vi "LC_BESS_Main.vi"() -> ()   [LabVIEW 2016]
uses:
  LabVIEW Data/MathScriptVIs/MCStatic_36913153632_b27534ebdc28079805a0f770a8a2da2a.vi
  <instcachedir>/0/MCStatic_36913153632_b27534ebdc28079805a0f770a8a2da2a_943E3674364E42B8AD23C55717B072BE.lvgen/MCStatic_36913153632_b27534ebdc28079805a0f770a8a2da2a_943E3674364E42B8AD23C55717B072BE_000.vi
  <vilib>/imath/engines/lvmath2/RunTimeEngine/BuiltInFunctions/abs/NIMS_abs(unsigned).vi
  <instcachedir>/0/NIMS_abs(unsigned)_CB0E2CC90712458C87FBF103B22FBEA1.lvgen/NIMS_abs(unsigned)_CB0E2CC90712458C87FBF103B22FBEA1_002.vi
  <vilib>/imath/engines/lvmath2/RunTimeEngine/NodeEndStatement/NIMS_NodeEndStatement_Output.vi
  <instcachedir>/0/NIMS_NodeEndStatement_Output_53EC0D466D134D7ABD903AC30B43404B.lvgen/NIMS_NodeEndStatement_Output_53EC0D466D134D7ABD903AC30B43404B_001.vi
  <vilib>/imath/engines/lvmath2/RunTimeEngine/ErrorHandling/NIMS_Finalize Error.vi
  <vilib>/ErrorRing/Error Ring.xnode
  BESS_LC/PIcontroller.m
panel:
  out "Waveform Chart":dbl[][](graph)=[[-0.0, 0.25, 0.0]]
  in  "BESS_Active_Power_Cmd 2":fxp<+/-,64,32>=0.25
  out "MGCC_to_BESS":dbl[](array[numeric])=[1.0, 0.0, 0.0, 0.0, 0.0, 0.0, 0.0] format="%#_6f"
  in  "p_mag":dbl=-1.0
  in  "i_mag":dbl=-1.0
  out "Waveform Chart 2":dbl(graph)
  out "BESS_Start_Stop_Cmd":bool
  out "error out 3":errorcluster
  out "error out 2":errorcluster
  out "BESS_Active_Power_Cmd":fxp<+/-,64,32>=0.25
  in  "Enable":bool=TRUE
  in  "p_in":dbl=0.5
  in  "i_in":dbl=0.2
  in  "p_an":dbl=0.2
  in  "i_an":dbl=0.05
  out "error out":errorcluster
  in  "BESS_Start_Stop":bool
  in  "BESS_Rective_Power_Cmd":fxp<+/-,64,32>=-1.0
  out "BESS_F":fxp<+/-,64,32>=59.92425537109375
  out "BESS_P":fxp<+/-,64,32>=0.000335693359375
  out "BESS_Q":fxp<+/-,64,32>=0.0039520263671875
  out "BESS_V":fxp<+/-,64,32>=0.0112762451171875
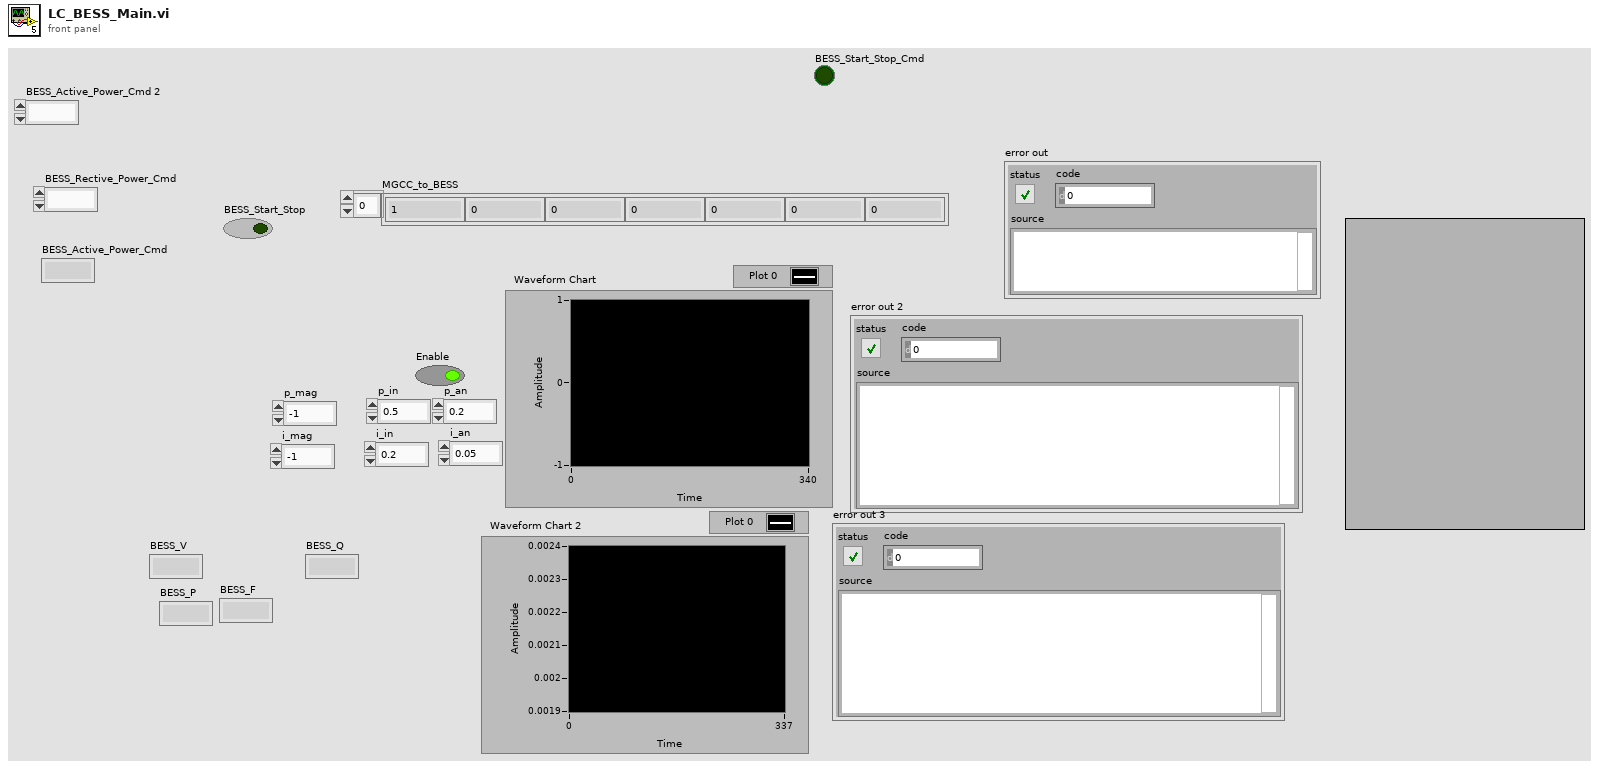
[diagram p1: front panel]
types:
  T1 = typedef "NI_Matrix.lvlib/RealMatrix.ctl" = dbl[][]
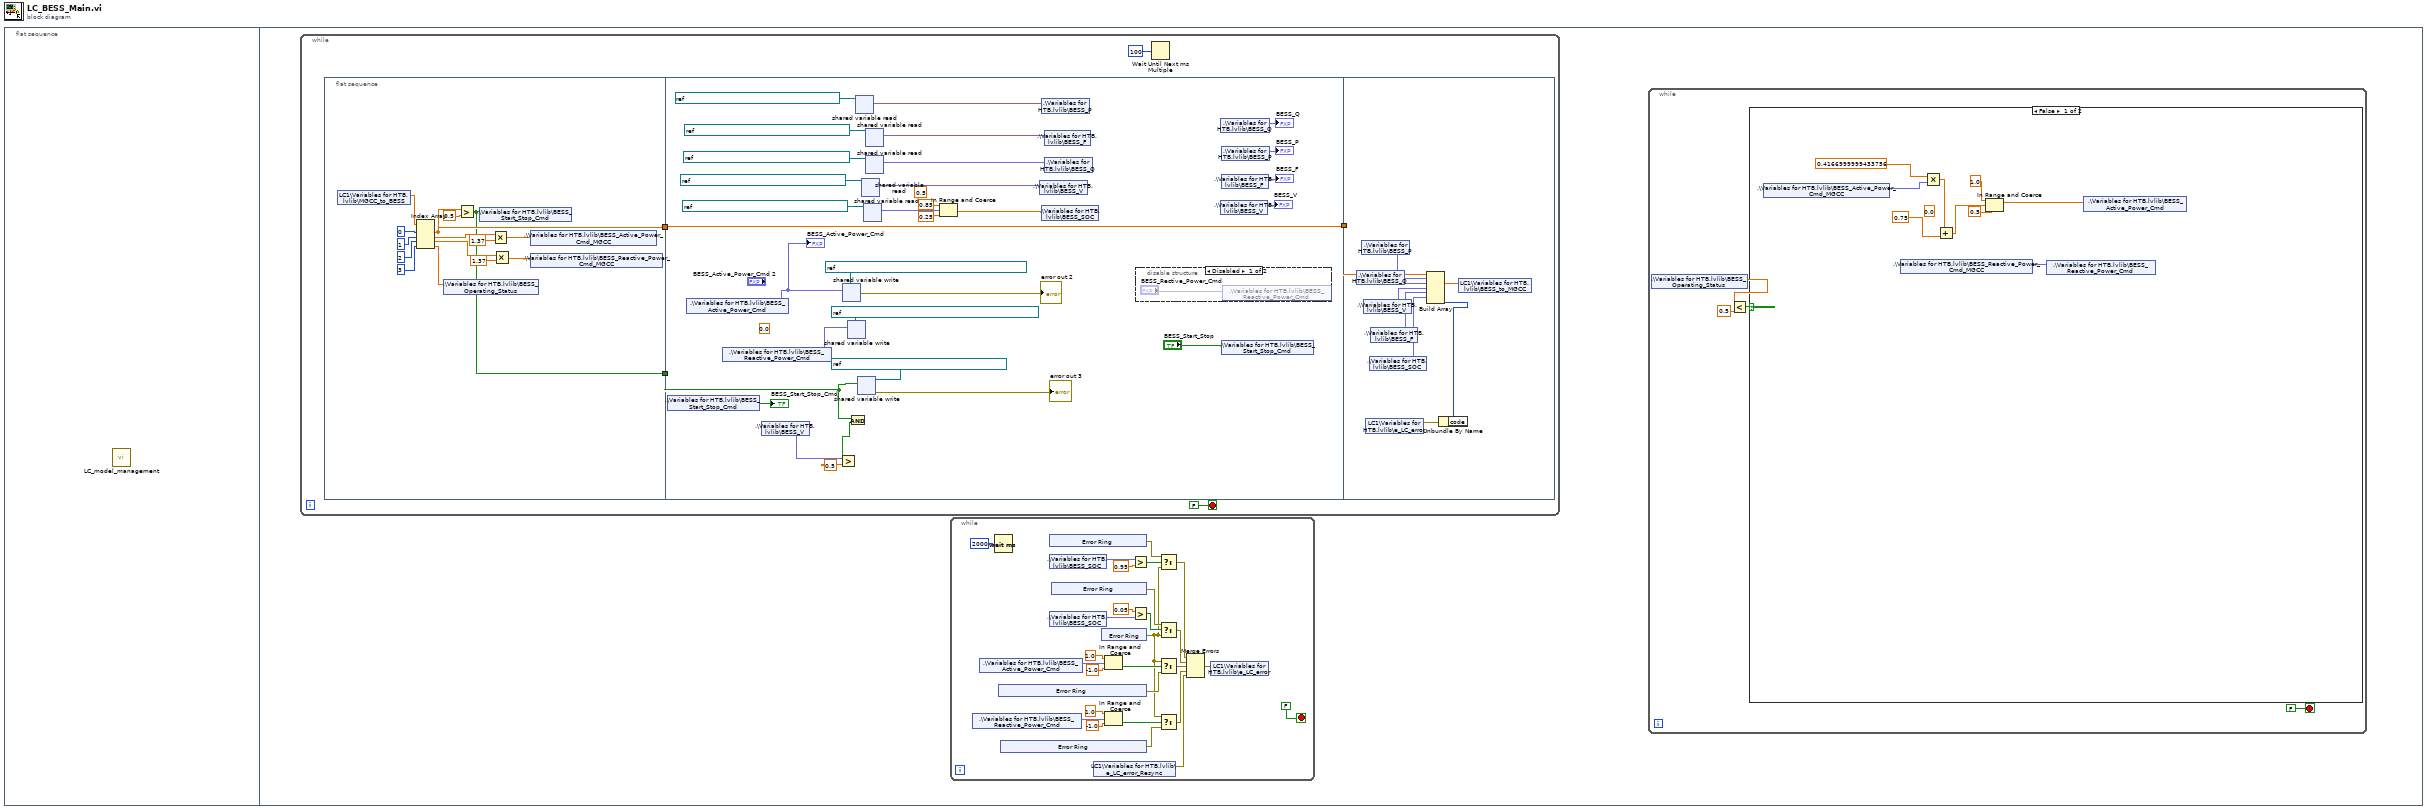
[diagram p0: block diagram]
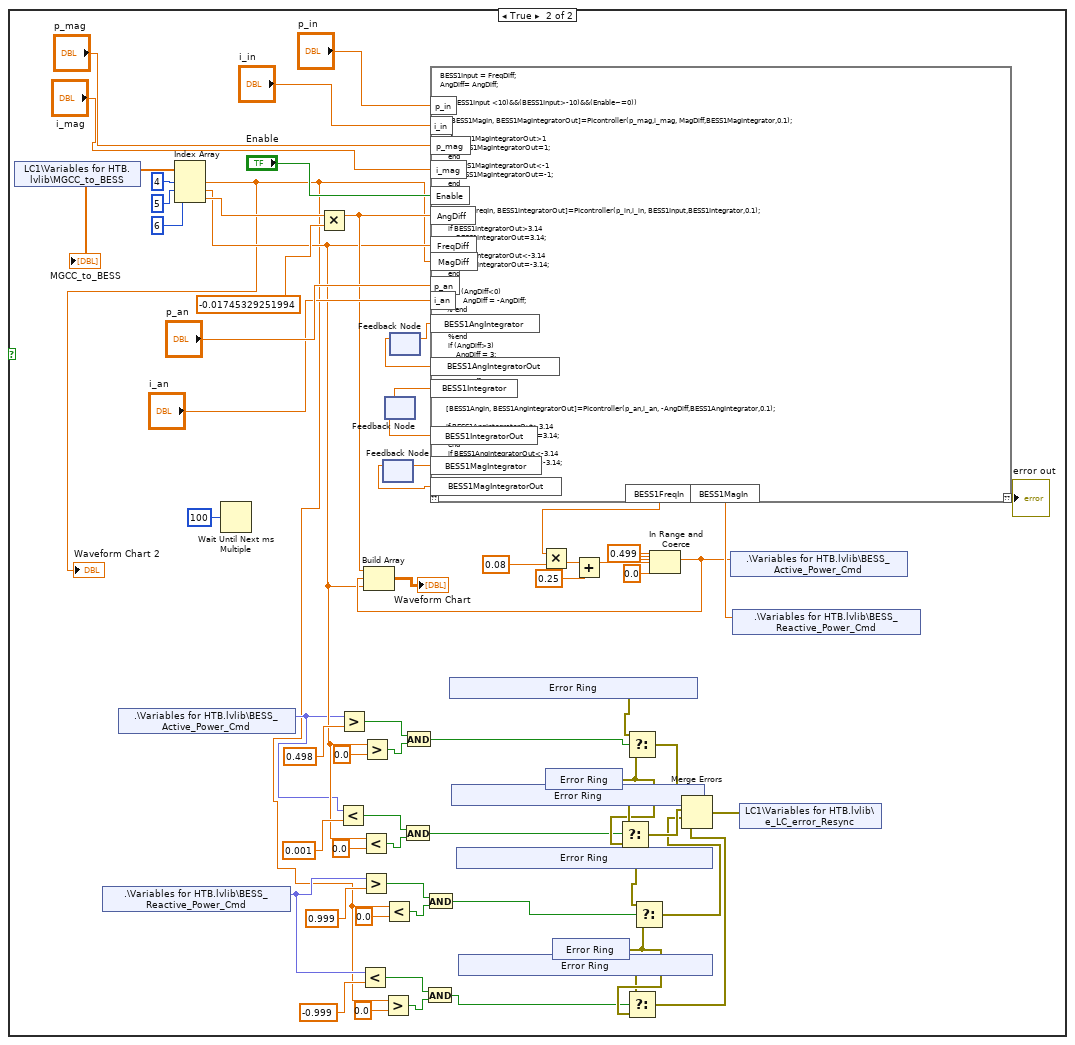
[diagram p2: hidden frame]
diagram:
  n1 = flat-sequence {
    frame #0 {
      n2 = call "LC_model_management.vi"() -> ()  [unwired: 12 in]
    }
    frame #1 {
      n3 = while {
        stop <- FALSE stop-if-true
        n4 = flat-sequence {
          tunnel: [w586] -> w573
          tunnel: [w583] -> w572
          tunnel: [w609] -> w574
          tunnel: w573 -> [w609]
          tunnel: w572 -> [w605]
          tunnel: w574 -> [w626]
          frame #0 {
            n5 = shared-variable "LC1\\Variables for HTB.lvlib\\MGCC_to_BESS"() -> (w591:dbl[])  [unwired: 1 in, 1 out]
            n6 = Index Array(array=w591, index #1=0 ("index"), index #2=1 ("index"), index #3=2 ("index"), index #4=3 ("index")) -> (element #1=w586:dbl, element #2=w582:dbl, element #3=w578:dbl, element #4=w584:dbl)
            n7 = shared-variable ".\\Variables for HTB.lvlib\\BESS_Operating_Status"(w584) -> ()  [unwired: 1 in, 1 out]
            n8 = Greater?(x=w586, y=0.5) -> (0:w583:bool)
            n9 = shared-variable ".\\Variables for HTB.lvlib\\BESS_Start_Stop_Cmd"(w583) -> ()  [unwired: 1 in, 1 out]
            n10 = Multiply(x=w582, y=1.37) -> (x*y=w581:dbl)
            n11 = Multiply(x=w578, y=1.37) -> (x*y=w579:dbl)
            n12 = shared-variable ".\\Variables for HTB.lvlib\\BESS_Active_Power_Cmd_MGCC"(w581) -> ()  [unwired: 1 in, 1 out]
            n13 = shared-variable ".\\Variables for HTB.lvlib\\BESS_Reactive_Power_Cmd_MGCC"(w579) -> ()  [unwired: 1 in, 1 out]
          }
          frame #1 {
            (unwired) 0.5
            (unwired) 0.0 ("lower limit")
            n14 = shared-variable ".\\Variables for HTB.lvlib\\BESS_Start_Stop_Cmd"() -> (→"BESS_Start_Stop_Cmd":bool)  [unwired: 1 in, 1 out]
            n15 = shared-variable ".\\Variables for HTB.lvlib\\BESS_Active_Power_Cmd"() -> (w594:fxp<+/-,64,32>)  [unwired: 1 in, 1 out]
            "BESS_Active_Power_Cmd" <- w594
            n16 = shared-variable ".\\Variables for HTB.lvlib\\BESS_Reactive_Power_Cmd"() -> (w593:fxp<+/-,64,32>)  [unwired: 1 in, 1 out]
            n17 = shared-variable ".\\Variables for HTB.lvlib\\BESS_V"() -> (w601:fxp<+/-,64,32>)  [unwired: 1 in, 1 out]
            n18 = Greater?(x=w601, y=0.5) -> (0:w606:bool)
            n19 = shared-variable-write(refnum<k21> "ni.var.psp://cepd00622/Variables from Host/L1 Active Power" ("shared variable refnum in"), w594) -> (→"error out 2":errorcluster)  [unwired: 1 in, 1 out]
            n20 = shared-variable-write(refnum<k21> "ni.var.psp://cepd00622/Variables from Host/L1 Reactive Power" ("shared variable refnum in"), w593) -> ()  [unwired: 1 in, 2 out]
            n21 = And(x=w605, y=w606) -> ()  [unwired: 1 out]
            n22 = shared-variable-read(refnum<k21> "ni.var.psp://cepd00622/Variables from Host/L1 P" ("shared variable refnum in")) -> (w612:fxp<+/-,64,32>)  [unwired: 1 in, 2 out]
            n23 = shared-variable-write(refnum<k21> "ni.var.psp://cepd00622/Variables from Host/L1 Start" ("shared variable refnum in"), w605) -> (→"error out 3":errorcluster)  [unwired: 1 in, 1 out]
            n24 = shared-variable-read(refnum<k21> "ni.var.psp://cepd00622/Variables from Host/L1 V" ("shared variable refnum in")) -> (w617:fxp<+/-,64,32>)  [unwired: 1 in, 2 out]
            n25 = shared-variable-read(refnum<k21> "ni.var.psp://cepd00622/Variables from Host/L8 V" ("shared variable refnum in")) -> (w595:fxp<+/-,64,32>)  [unwired: 1 in, 2 out]
            n26 = shared-variable-read(refnum<k21> "ni.var.psp://cepd00622/Variables from Host/L1 F" ("shared variable refnum in")) -> (w600:fxp<+/-,64,32>)  [unwired: 1 in, 2 out]
            n27 = shared-variable-read(refnum<k21> "ni.var.psp://cepd00622/Variables from Host/L1 Q" ("shared variable refnum in")) -> (w614:fxp<+/-,64,32>)  [unwired: 1 in, 2 out]
            n28 = In Range and Coerce(upper limit=0.85, x=w595, lower limit=0.25) -> (coerced(x)=w592:dbl)  [unwired: 1 out]
            n29 = shared-variable ".\\Variables for HTB.lvlib\\BESS_V"(w617) -> ()  [unwired: 1 in, 1 out]
            n30 = shared-variable ".\\Variables for HTB.lvlib\\BESS_P"(w612) -> ()  [unwired: 1 in, 1 out]
            n31 = shared-variable ".\\Variables for HTB.lvlib\\BESS_SOC"(w592) -> ()  [unwired: 1 in, 1 out]
            n32 = shared-variable ".\\Variables for HTB.lvlib\\BESS_F"(w600) -> ()  [unwired: 1 in, 1 out]
            n33 = shared-variable ".\\Variables for HTB.lvlib\\BESS_Q"(w614) -> ()  [unwired: 1 in, 1 out]
            n34 = disable-structure shown="Disabled" {
              frame Disabled {
                n35 = shared-variable ".\\Variables for HTB.lvlib\\BESS_Reactive_Power_Cmd"("BESS_Rective_Power_Cmd") -> ()  [unwired: 1 in, 1 out]
              }
              frame Enabled {
              }
            }
            n36 = shared-variable ".\\Variables for HTB.lvlib\\BESS_Q"() -> (→"BESS_Q":fxp<+/-,64,32>)  [unwired: 1 in, 1 out]
            n37 = shared-variable ".\\Variables for HTB.lvlib\\BESS_V"() -> (→"BESS_V":fxp<+/-,64,32>)  [unwired: 1 in, 1 out]
            n38 = shared-variable ".\\Variables for HTB.lvlib\\BESS_P"() -> (→"BESS_P":fxp<+/-,64,32>)  [unwired: 1 in, 1 out]
            n39 = shared-variable ".\\Variables for HTB.lvlib\\BESS_F"() -> (→"BESS_F":fxp<+/-,64,32>)  [unwired: 1 in, 1 out]
            n40 = shared-variable ".\\Variables for HTB.lvlib\\BESS_Start_Stop_Cmd"("BESS_Start_Stop") -> ()  [unwired: 1 in, 1 out]
          }
          frame #2 {
            n41 = shared-variable ".\\Variables for HTB.lvlib\\BESS_Q"() -> (w631:fxp<+/-,64,32>)  [unwired: 1 in, 1 out]
            n42 = shared-variable ".\\Variables for HTB.lvlib\\BESS_P"() -> (w632:fxp<+/-,64,32>)  [unwired: 1 in, 1 out]
            n43 = shared-variable ".\\Variables for HTB.lvlib\\BESS_V"() -> (w630:fxp<+/-,64,32>)  [unwired: 1 in, 1 out]
            n44 = shared-variable "LC1\\Variables for HTB.lvlib\\e_LC_error"() -> (w625:errorcluster)  [unwired: 1 in, 1 out]
            n45 = shared-variable ".\\Variables for HTB.lvlib\\BESS_SOC"() -> (w627:fxp<+/-,64,32>)  [unwired: 1 in, 1 out]
            n46 = shared-variable ".\\Variables for HTB.lvlib\\BESS_F"() -> (w629:fxp<+/-,64,32>)  [unwired: 1 in, 1 out]
            n47 = Unbundle By Name(w625) -> ("code"=w624:i32)
            n48 = Build Array(w626, w632, w631, w630, w629, w627, w624) -> (w628:dbl[])
            n49 = shared-variable "LC1\\Variables for HTB.lvlib\\BESS_to_MGCC"(w628) -> ()  [unwired: 1 in, 1 out]
          }
        }
        n50 = Wait Until Next ms Multiple(millisecond multiple=u32 100 ("milliseconds to wait")) -> ()  [unwired: 1 out]
      }
      n51 = while {
        stop <- FALSE stop-if-true
        n52 = shared-variable ".\\Variables for HTB.lvlib\\BESS_Reactive_Power_Cmd"() -> (w2:fxp<+/-,64,32>)  [unwired: 1 in, 1 out]
        n53 = shared-variable ".\\Variables for HTB.lvlib\\BESS_Active_Power_Cmd"() -> (w12:fxp<+/-,64,32>)  [unwired: 1 in, 1 out]
        n54 = Wait (ms)(milliseconds to wait=u32 2000) -> ()  [unwired: 1 out]
        n55 = xnode "Error Ring"() -> ("error out"=w10:errorcluster)
        n56 = xnode "Error Ring"() -> ("error out"=w5:errorcluster)
        n57 = xnode "Error Ring"() -> ("error out"=w21:errorcluster)
        n58 = shared-variable ".\\Variables for HTB.lvlib\\BESS_SOC"() -> (w25:fxp<+/-,64,32>)  [unwired: 1 in, 1 out]
        n59 = shared-variable ".\\Variables for HTB.lvlib\\BESS_SOC"() -> (w18:fxp<+/-,64,32>)  [unwired: 1 in, 1 out]
        n60 = xnode "Error Ring"() -> ("error out"=w16:errorcluster)
        n61 = shared-variable "LC1\\Variables for HTB.lvlib\\e_LC_error_Resync"() -> (w1:errorcluster)  [unwired: 1 in, 1 out]
        n62 = xnode "Error Ring"() -> ("error out"=w4:errorcluster)
        n63 = In Range and Coerce(upper limit=1.0, x=w12, lower limit=-1.0) -> (In Range?=w11:bool)  [unwired: 1 out]
        n64 = In Range and Coerce(upper limit=1.0, x=w2, lower limit=-1.0) -> (In Range?=w8:bool)  [unwired: 1 out]
        n65 = Greater?(x=w25, y=0.95 ("upper limit")) -> (0:w22:bool)
        n66 = Greater?(x=0.05 ("lower limit"), y=w18) -> (0:w17:bool)
        n67 = Select(t=w21, s=w22, f=w4) -> (s? t:f=w20:errorcluster)
        n68 = Select(t=w16, s=w17, f=w4) -> (s? t:f=w15:errorcluster)
        n69 = Select(t=w4, s=w11, f=w10) -> (s? t:f=w9:errorcluster)
        n70 = Select(t=w4, s=w8, f=w5) -> (s? t:f=w3:errorcluster)
        n71 = Merge Errors(w20, w15, w9, w3, w1) -> (w23:errorcluster)
        n72 = shared-variable "LC1\\Variables for HTB.lvlib\\e_LC_error"(w23) -> ()  [unwired: 1 in, 1 out]
      }
      n73 = while {
        stop <- FALSE stop-if-true
        n74 = shared-variable ".\\Variables for HTB.lvlib\\BESS_Operating_Status"() -> (w35:dbl)  [unwired: 1 in, 1 out]
        n75 = Less?(x=w35, y=0.5) -> (x < y?=w33:bool)
        n76 = case shown="False" w33 {
          frame False {
            (unwired) 0.0 ("x")
            n77 = shared-variable ".\\Variables for HTB.lvlib\\BESS_Active_Power_Cmd_MGCC"() -> (w41:fxp<+/-,64,32>)  [unwired: 1 in, 1 out]
            n78 = shared-variable ".\\Variables for HTB.lvlib\\BESS_Reactive_Power_Cmd_MGCC"() -> (w39:fxp<+/-,64,32>)  [unwired: 1 in, 1 out]
            n79 = Multiply(x=0.4166999999433756 ("BESS_Active_Power_Cmd"), y=w41) -> (x*y=w38:dbl)
            n80 = Add(x=w38, y=0.75 ("BESS_Active_Power_Cmd")) -> (x+y=w43:dbl)
            n81 = In Range and Coerce(upper limit=1.0, x=w43, lower limit=0.5) -> (coerced(x)=w37:dbl)  [unwired: 1 out]
            n82 = shared-variable ".\\Variables for HTB.lvlib\\BESS_Reactive_Power_Cmd"(w39) -> ()  [unwired: 1 in, 1 out]
            n83 = shared-variable ".\\Variables for HTB.lvlib\\BESS_Active_Power_Cmd"(w37) -> ()  [unwired: 1 in, 1 out]
          }
          frame True {
            n84 = shared-variable "LC1\\Variables for HTB.lvlib\\MGCC_to_BESS"() -> (w94:dbl[])  [unwired: 1 in, 1 out]
            "MGCC_to_BESS" <- w94
            n85 = shared-variable ".\\Variables for HTB.lvlib\\BESS_Reactive_Power_Cmd"() -> (w54:fxp<+/-,64,32>)  [unwired: 1 in, 1 out]
            n86 = shared-variable ".\\Variables for HTB.lvlib\\BESS_Active_Power_Cmd"() -> (w55:fxp<+/-,64,32>)  [unwired: 1 in, 1 out]
            n87 = Index Array(array=w94, index #1=4 ("index"), index #2=5 ("index"), index #3=6 ("index")) -> (element #1=w53:dbl, element #2=w65:dbl, element #3=w90:dbl)
            "Waveform Chart 2" <- w53
            n88 = Wait Until Next ms Multiple(millisecond multiple=u32 100) -> ()  [unwired: 1 out]
            n89 = Multiply(x=w90, y=-0.01745329251994) -> (x*y=w82:dbl)
            n90 = Less?(x=w55, y=0.001 ("upper limit")) -> (x < y?=w67:bool)
            n91 = Greater?(x=w55, y=0.498 ("upper limit")) -> (0:w79:bool)
            n92 = Less?(x=w54, y=-0.999 ("upper limit")) -> (x < y?=w62:bool)
            n93 = Less?(x=w65, y=0.0) -> (x < y?=w69:bool)
            n94 = Greater?(x=w54, y=0.999 ("upper limit")) -> (0:w57:bool)
            n95 = Greater?(x=w65, y=0.0) -> (0:w77:bool)
            n96 = feedback #1() -> (w85:dbl)  [unwired: 1 in]
            n97 = Greater?(x=w53, y=0.0) -> (0:w60:bool)
            n98 = Less?(x=w53, y=0.0) -> (x < y?=w59:bool)
            n99 = feedback #2() -> (w112:dbl)  [unwired: 1 in]
            n100 = feedback #3() -> (w109:dbl)  [unwired: 1 in]
            n101 = And(x=w67, y=w69) -> (x .and. y?=w64:bool)
            n102 = And(x=w79, y=w77) -> (x .and. y?=w70:bool)
            n103 = And(x=w62, y=w60) -> (x .and. y?=w46:bool)
            n104 = And(x=w57, y=w59) -> (x .and. y?=w47:bool)
            n105 = mathscript code="BESS1Input = FreqDiff;\nAngDiff= AngDiff;\n\nif ((BESS1Input <10)&&(BESS1Input>-10)&&(Enable~=0))\n\n    [BESS1MagIn, BESS1MagIntegratorOut]=PIcontroller(p_mag,i_mag, MagDiff,BESS1MagIntegrator,0.1);\n   \n    if BESS1MagIntegratorOut>1\n        BESS1MagIntegratorOut=1;\n    end\n    if BESS1MagIntegratorOut<-1\n        BESS1MagIntegratorOut=-1;\n    end\n\n\n    [BESS1FreqIn, BESS1IntegratorOut]=PIcontroller(p_in,i_in, BESS1Input,BESS1Integrator,0.1);\n   \n    if BESS1IntegratorOut>3.14\n        BESS1IntegratorOut=3.14;\n    end\n    if BESS1IntegratorOut<-3.14\n        BESS1IntegratorOut=-3.14;\n    end\n\n%    if (AngDiff<0)\n %       AngDiff = -AngDiff;\n   % end \n    %if (AngDiff> 5)\n     %   AngDiff = 0;\n    %end \n    if (AngDiff>3)\n        AngDiff = 3;\n    end \n    if (AngDiff<-3)\n        AngDiff = -3;\n    end \n\n   [BESS1AngIn, BESS1AngIntegratorOut]=PIcontroller(p_an,i_an, -AngDiff,BESS1AngIntegrator,0.1);\n\n   if BESS1AngIntegratorOut>3.14\n        BESS1AngIntegratorOut=3.14;\n    end\n    if BESS1AngIntegratorOut<-3.14\n        BESS1AngIntegratorOut=-3.14;\n    end\n    \n    if abs(FreqDiff<0.2)\n        BESS1FreqIn = BESS1FreqIn + BESS1AngIn;\n    else\n        BESS1AngIntegratorOut = 0;\n    end\n    if (BESS1FreqIn > 3.14) \n          BESS1FreqIn = 3.14;\n    end\n    if (BESS1FreqIn < -3.14) \n          BESS1FreqIn = -3.14;\n    end\n\n    if (AngDiff ==0)&&(FreqDiff == 0) && (MagDiff== 0)\n        BESS1FreqIn = 0;\n        BESS1MagIn = 0;\n        BESS1IntegratorOut = 0;\n        BESS1MagIntegratorOut = 0;\n        BESS1AngIntegratorOut = 0;\n    end\n\nelse\nBESS1FreqIn = 0;\nBESS1MagIn = 0;\nBESS1IntegratorOut = 0;\nBESS1MagIntegratorOut = 0;\nBESS1AngIntegratorOut = 0;\nend"("AngDiff"=w82, "BESS1Integrator"=w112, "FreqDiff"=w65, "BESS1AngIntegrator"=w109, "Enable"="Enable", "p_in"="p_in", "i_in"="i_in", "p_an"="p_an", "i_an"="i_an", "p_mag"="p_mag", "i_mag"="i_mag", "BESS1MagIntegrator"=w85, "MagDiff"=w53) -> ("??"=→"error out":errorcluster, "BESS1IntegratorOut"=w111:dbl, "BESS1FreqIn"=w86:dbl, "BESS1AngIntegratorOut"=w110:dbl, "BESS1MagIntegratorOut"=w87:dbl, "BESS1MagIn"=w84:dbl)  [unwired: 1 in]
            n106 = feedback-in #1(w87) -> ()
            n107 = feedback-in #2(w111) -> ()
            n108 = feedback-in #3(w110) -> ()
            n109 = xnode "Error Ring"() -> ("error out"=w75:errorcluster)
            n110 = xnode "Error Ring"() -> ("error out"=w73:errorcluster)
            n111 = xnode "Error Ring"() -> ("error out"=w50:errorcluster)
            n112 = xnode "Error Ring"() -> ("error out"=w51:errorcluster)
            n113 = Multiply(x=w86, y=0.08 ("upper limit")) -> (x*y=w98:dbl)
            n114 = xnode "Error Ring"() -> ("error out"=w71:errorcluster)
            n115 = xnode "Error Ring"() -> ("error out"=w52:errorcluster)
            n116 = Add(x=w98, y=0.25) -> (x+y=w96:dbl)
            n117 = Select(t=w73, s=w64, f=w71) -> (s? t:f=w72:errorcluster)
            n118 = Select(t=w75, s=w70, f=w71) -> (s? t:f=w74:errorcluster)
            n119 = Select(t=w51, s=w46, f=w52) -> (s? t:f=w48:errorcluster)
            n120 = Select(t=w50, s=w47, f=w52) -> (s? t:f=w49:errorcluster)
            n121 = In Range and Coerce(upper limit=0.499, x=w96, lower limit=0.0) -> (coerced(x)=w81:dbl)  [unwired: 1 out]
            n122 = Build Array(w82, w81, w65) -> (→"Waveform Chart":T1)
            n123 = Merge Errors(w74, w72, w49, w48) -> (w76:errorcluster)
            n124 = shared-variable ".\\Variables for HTB.lvlib\\BESS_Active_Power_Cmd"(w81) -> ()  [unwired: 1 in, 1 out]
            n125 = shared-variable ".\\Variables for HTB.lvlib\\BESS_Reactive_Power_Cmd"(w84) -> ()  [unwired: 1 in, 1 out]
            n126 = shared-variable "LC1\\Variables for HTB.lvlib\\e_LC_error_Resync"(w76) -> ()  [unwired: 1 in, 1 out]
          }
        }
      }
    }
  }
